vi "Monty_Hall_Game_Premium[1].vi"() -> ()   [LabVIEW 2025]
uses:
  <vilib>/numeric/Random Number (Range) I64.vi
  <vilib>/numeric/sub_Random U32.vi
panel:
  in  "Number of doors":i32=1 min=3 max=10 step=1
  out "Boolean 10":bool
  out "Boolean 9":bool
  out "Boolean 8":bool
  out "Boolean 7":bool
  out "Boolean 6":bool
  out "Boolean 5":bool
  out "Boolean 4":bool
  out "Boolean 3":bool
  out "Boolean 2":bool
  out "Boolean":bool
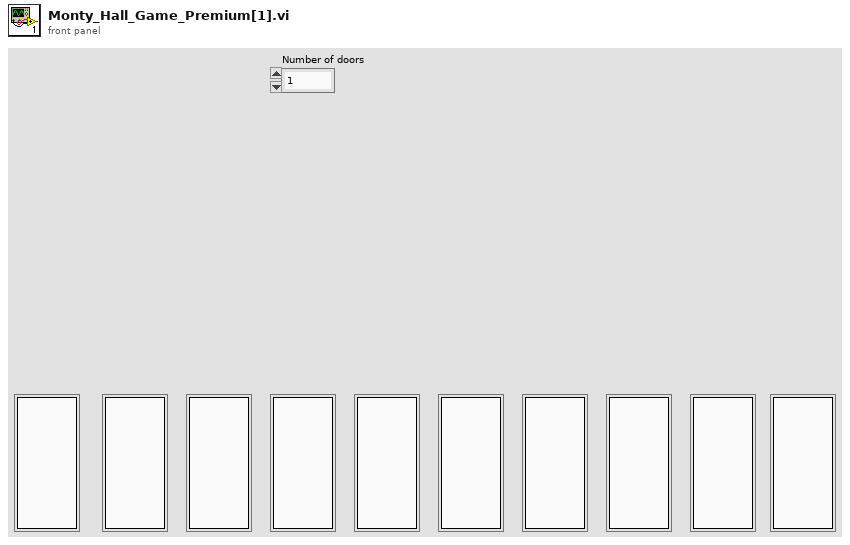
[diagram p1: front panel]
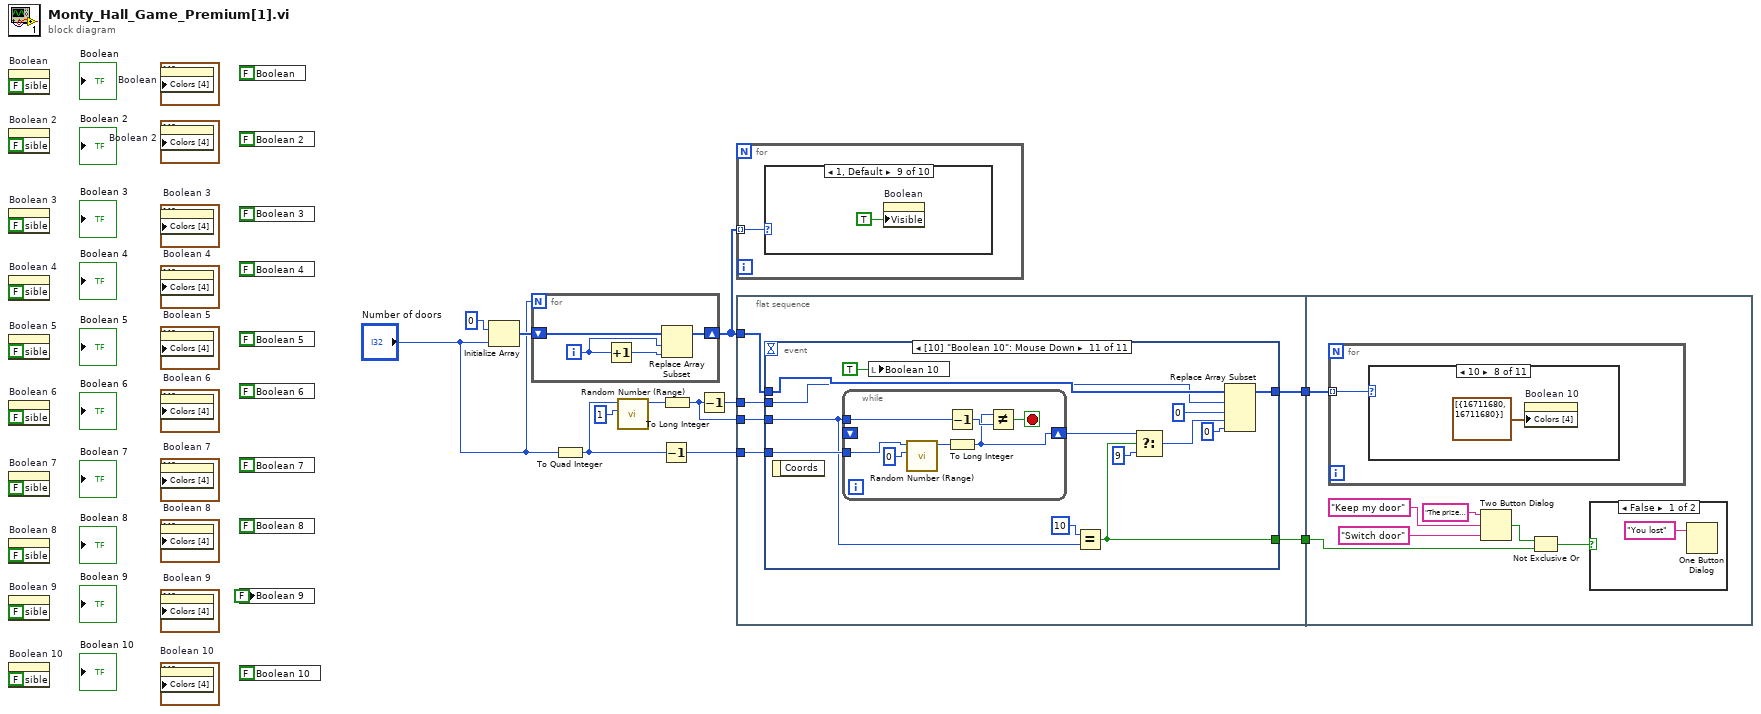
[diagram p0: block diagram]
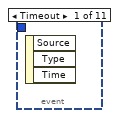
[diagram p2: hidden frame]
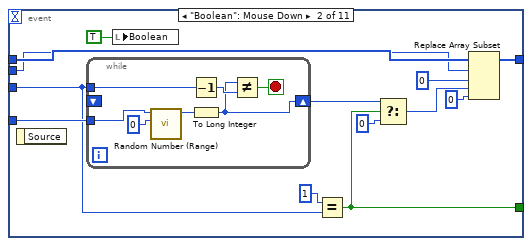
[diagram p3: hidden frame]
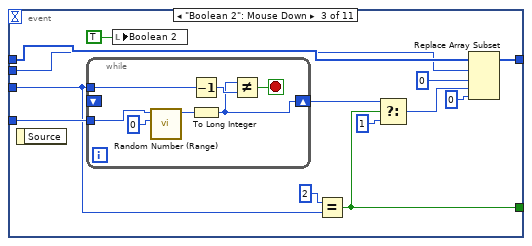
[diagram p4: hidden frame]
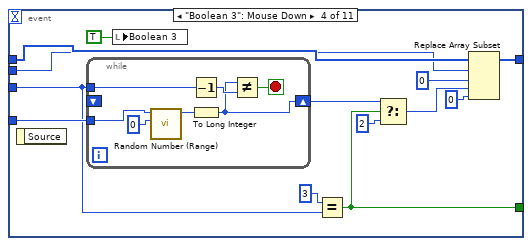
[diagram p5: hidden frame]
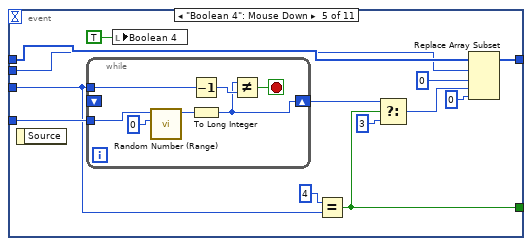
[diagram p6: hidden frame]
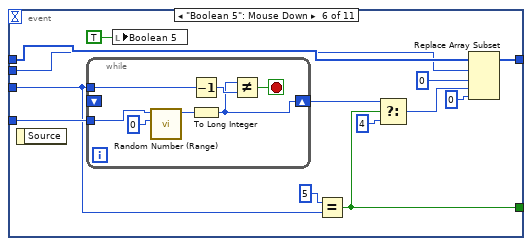
[diagram p7: hidden frame]
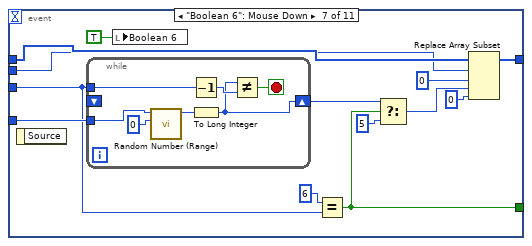
[diagram p8: hidden frame]
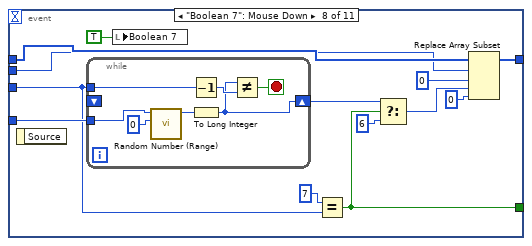
[diagram p9: hidden frame]
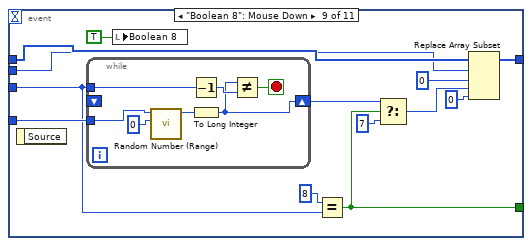
[diagram p10: hidden frame]
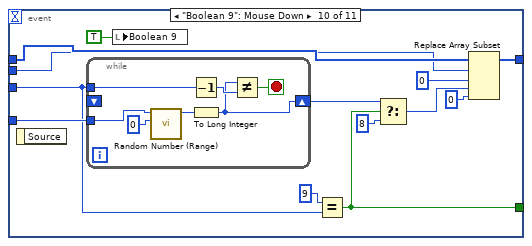
[diagram p11: hidden frame]
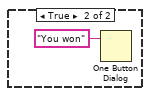
[diagram p12: hidden frame]
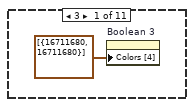
[diagram p13: hidden frame]
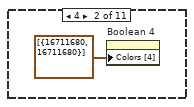
[diagram p14: hidden frame]
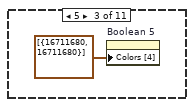
[diagram p15: hidden frame]
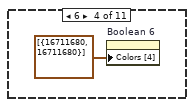
[diagram p16: hidden frame]
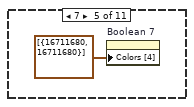
[diagram p17: hidden frame]
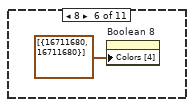
[diagram p18: hidden frame]
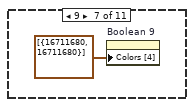
[diagram p19: hidden frame]
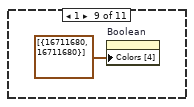
[diagram p20: hidden frame]
diagram:
  n1 = property on="Boolean" class="Bool (strict)"("Visible"=FALSE) -> ()  [unwired: 2 in, 2 out]
  n2 = property on="Boolean 2" class="Bool (strict)"("Visible"=FALSE) -> ()  [unwired: 2 in, 2 out]
  n3 = property on="Boolean 3" class="Bool (strict)"("Visible"=FALSE) -> ()  [unwired: 2 in, 2 out]
  n4 = property on="Boolean 4" class="Bool (strict)"("Visible"=FALSE) -> ()  [unwired: 2 in, 2 out]
  n5 = property on="Boolean 5" class="Bool (strict)"("Visible"=FALSE) -> ()  [unwired: 2 in, 2 out]
  n6 = property on="Boolean 6" class="Bool (strict)"("Visible"=FALSE) -> ()  [unwired: 2 in, 2 out]
  n7 = property on="Boolean 7" class="Bool (strict)"("Visible"=FALSE) -> ()  [unwired: 2 in, 2 out]
  n8 = property on="Boolean 8" class="Bool (strict)"("Visible"=FALSE) -> ()  [unwired: 2 in, 2 out]
  n9 = property on="Boolean 9" class="Bool (strict)"("Visible"=FALSE) -> ()  [unwired: 2 in, 2 out]
  n10 = property on="Boolean 10" class="Bool (strict)"("Visible"=FALSE) -> ()  [unwired: 2 in, 2 out]
  n11 = property on="Boolean" class="Bool (strict)"("Colors [4]"=cluster{u32, u32}[] [{0, 16448250}]) -> ()  [unwired: 2 in, 2 out]
  n12 = property on="Boolean 2" class="Bool (strict)"("Colors [4]"=cluster{u32, u32}[] [{0, 16448250}]) -> ()  [unwired: 2 in, 2 out]
  n13 = property on="Boolean 3" class="Bool (strict)"("Colors [4]"=cluster{u32, u32}[] [{0, 16448250}]) -> ()  [unwired: 2 in, 2 out]
  n14 = property on="Boolean 4" class="Bool (strict)"("Colors [4]"=cluster{u32, u32}[] [{0, 16448250}]) -> ()  [unwired: 2 in, 2 out]
  n15 = property on="Boolean 5" class="Bool (strict)"("Colors [4]"=cluster{u32, u32}[] [{0, 16448250}]) -> ()  [unwired: 2 in, 2 out]
  n16 = property on="Boolean 6" class="Bool (strict)"("Colors [4]"=cluster{u32, u32}[] [{0, 16448250}]) -> ()  [unwired: 2 in, 2 out]
  n17 = property on="Boolean 7" class="Bool (strict)"("Colors [4]"=cluster{u32, u32}[] [{0, 16448250}]) -> ()  [unwired: 2 in, 2 out]
  n18 = property on="Boolean 8" class="Bool (strict)"("Colors [4]"=cluster{u32, u32}[] [{0, 16448250}]) -> ()  [unwired: 2 in, 2 out]
  n19 = property on="Boolean 9" class="Bool (strict)"("Colors [4]"=cluster{u32, u32}[] [{0, 16448250}]) -> ()  [unwired: 2 in, 2 out]
  n20 = property on="Boolean 10" class="Bool (strict)"("Colors [4]"=cluster{u32, u32}[] [{0, 16448250}]) -> ()  [unwired: 2 in, 2 out]
  n21 = local write "Boolean"(FALSE ("Boolean")) -> ()
  n22 = local write "Boolean 2"(FALSE ("Boolean")) -> ()
  n23 = local write "Boolean 3"(FALSE ("Boolean")) -> ()
  n24 = local write "Boolean 4"(FALSE ("Boolean")) -> ()
  n25 = local write "Boolean 5"(FALSE ("Boolean")) -> ()
  n26 = local write "Boolean 6"(FALSE ("Boolean")) -> ()
  n27 = local write "Boolean 7"(FALSE ("Boolean")) -> ()
  n28 = local write "Boolean 8"(FALSE ("Boolean")) -> ()
  n29 = local write "Boolean 9"(FALSE ("Boolean")) -> ()
  n30 = local write "Boolean 10"(FALSE ("Boolean")) -> ()
  n31 = Initialize Array(0 ("element"), "Number of doors") -> (w41:i32[])
  n32 = for {
    N: "Number of doors" -> [_]
    shift-right: [w43] -> w28
    shift-left: w41 -> [w46]
    i -> [w45]
    n33 = Increment(x=w45) -> (x+1=w44:i32)
    n34 = Replace Array Subset(array=w46, new element=w44, index=w45) -> (w43:i32[])
  }
  n35 = To Quad Integer(1:"Number of doors") -> (0:w24:i64)
  n36 = call-poly <vilib>:"Random Number (Range).vi"("lower bound (-100)"=i64 1, "upper bound (100)"=w24) -> ("number"=w27:i64)  [unwired: 9 in]
  n37 = Decrement(x=w24) -> (x-1=w23:i64)
  n38 = To Long Integer(number=w27) -> (32bit integer=w26:i32)
  n39 = Decrement(x=w26) -> (x-1=w25:i32)
  n40 = for {
    tunnel: w28 -> [w47] mode=indexing
    n41 = case shown="1, Default" w47 {
      frame 3 {
        n42 = property on="Boolean 3" class="Bool (strict)"("Visible"=TRUE ("Boolean 4")) -> ()  [unwired: 2 in, 2 out]
      }
      frame 4 {
        n43 = property on="Boolean 4" class="Bool (strict)"("Visible"=TRUE) -> ()  [unwired: 2 in, 2 out]
      }
      frame 5 {
        n44 = property on="Boolean 5" class="Bool (strict)"("Visible"=TRUE) -> ()  [unwired: 2 in, 2 out]
      }
      frame 6 {
        n45 = property on="Boolean 6" class="Bool (strict)"("Visible"=TRUE) -> ()  [unwired: 2 in, 2 out]
      }
      frame 7 {
        n46 = property on="Boolean 7" class="Bool (strict)"("Visible"=TRUE) -> ()  [unwired: 2 in, 2 out]
      }
      frame 8 {
        n47 = property on="Boolean 8" class="Bool (strict)"("Visible"=TRUE) -> ()  [unwired: 2 in, 2 out]
      }
      frame 9 {
        n48 = property on="Boolean 9" class="Bool (strict)"("Visible"=TRUE) -> ()  [unwired: 2 in, 2 out]
      }
      frame 10 {
        n49 = property on="Boolean 10" class="Bool (strict)"("Visible"=TRUE) -> ()  [unwired: 2 in, 2 out]
      }
      frame 1, Default {
        n50 = property on="Boolean" class="Bool (strict)"("Visible"=TRUE) -> ()  [unwired: 2 in, 2 out]
      }
      frame 2 {
        n51 = property on="Boolean 2" class="Bool (strict)"("Visible"=TRUE ("Boolean 4")) -> ()  [unwired: 2 in, 2 out]
      }
    }
  }
  n52 = flat-sequence {
    tunnel: w28 -> [w63]
    tunnel: w26 -> [w62]
    tunnel: w25 -> [w61]
    tunnel: w23 -> [w60]
    tunnel: [w59] -> w22
    tunnel: [w58] -> w1
    tunnel: w22 -> [w270]
    tunnel: w1 -> [w267]
    frame #0 {
      n53 = event shown="[10] \"Boolean 10\": Mouse Down" {
        selector: _ -> [_ _ _ _ _ _ _ _ _ _ _]
        dyn-events: _ -> [_ _ _ _ _ _ _ _ _ _ _]
        timeout: _ -> [_ _ _ _ _ _ _ _ _ _ _]
        tunnel: w63 -> [_ w74 w90 w110 w130 w150 w170 w190 w210 w230 w250]
        tunnel: w62 -> [_ w69 w87 w107 w127 w147 w167 w187 w207 w227 w247]
        tunnel: w61 -> [_ w65 w89 w109 w129 w149 w169 w189 w209 w229 w249]
        tunnel: w60 -> [_ w70 w88 w108 w128 w148 w168 w188 w208 w228 w248]
        tunnel: [_ w67 w86 w106 w126 w146 w166 w186 w206 w226 w246] -> w59
        tunnel: [_ w64 w84 w104 w124 w144 w164 w184 w204 w224 w244] -> w58
        event Timeout {
          n54 = event-data() -> ()  [unwired: 1 in, 3 out]
        }
        event "Boolean": Mouse Down {
          n55 = event-data() -> ()  [unwired: 1 in, 1 out]
          n56 = while {
            tunnel: w70 -> [w81]
            tunnel: w69 -> [w79]
            shift-right: [w77] -> w68
            shift-left: _ -> [_]
            stop <- w78 stop-if-true
            n57 = call-poly <vilib>:"Random Number (Range).vi"("lower bound (-100)"=i64 0, "upper bound (100)"=w81) -> ("number"=w83:i64)  [unwired: 9 in]
            n58 = Decrement(x=w79) -> (x-1=w80:i32)
            n59 = To Long Integer(number=w83) -> (32bit integer=w77:i32)
            n60 = Not Equal?(x=w77, y=w80) -> (x != y?=w78:bool)
          }
          n61 = local write "Boolean"(TRUE ("Boolean")) -> ()
          n62 = Equal?(x=1, y=w69) -> (x = y?=w64:bool)
          n63 = Select(t=w68, s=w64, f=0 ("x")) -> (s? t:f=w72:i32)
          n64 = Replace Array Subset(array=w74, new element #1=0 ("new element/subarray"), index #1=w65, new element #2=0 ("new element/subarray"), index #2=w72) -> (w67:i32[])
        }
        event "Boolean 2": Mouse Down {
          n65 = event-data() -> ()  [unwired: 1 in, 1 out]
          n66 = while {
            tunnel: w88 -> [w101]
            tunnel: w87 -> [w99]
            shift-right: [w97] -> w91
            shift-left: _ -> [_]
            stop <- w98 stop-if-true
            n67 = call-poly <vilib>:"Random Number (Range).vi"("lower bound (-100)"=i64 0, "upper bound (100)"=w101) -> ("number"=w103:i64)  [unwired: 9 in]
            n68 = Decrement(x=w99) -> (x-1=w100:i32)
            n69 = To Long Integer(number=w103) -> (32bit integer=w97:i32)
            n70 = Not Equal?(x=w97, y=w100) -> (x != y?=w98:bool)
          }
          n71 = local write "Boolean 2"(TRUE ("Boolean")) -> ()
          n72 = Equal?(x=2, y=w87) -> (x = y?=w84:bool)
          n73 = Select(t=w91, s=w84, f=1 ("x")) -> (s? t:f=w93:i32)
          n74 = Replace Array Subset(array=w90, new element #1=0 ("new element/subarray"), index #1=w89, new element #2=0 ("new element/subarray"), index #2=w93) -> (w86:i32[])
        }
        event "Boolean 3": Mouse Down {
          n75 = event-data() -> ()  [unwired: 1 in, 1 out]
          n76 = while {
            tunnel: w108 -> [w121]
            tunnel: w107 -> [w119]
            shift-right: [w117] -> w111
            shift-left: _ -> [_]
            stop <- w118 stop-if-true
            n77 = call-poly <vilib>:"Random Number (Range).vi"("lower bound (-100)"=i64 0, "upper bound (100)"=w121) -> ("number"=w123:i64)  [unwired: 9 in]
            n78 = Decrement(x=w119) -> (x-1=w120:i32)
            n79 = To Long Integer(number=w123) -> (32bit integer=w117:i32)
            n80 = Not Equal?(x=w117, y=w120) -> (x != y?=w118:bool)
          }
          n81 = local write "Boolean 3"(TRUE ("Boolean")) -> ()
          n82 = Equal?(x=3, y=w107) -> (x = y?=w104:bool)
          n83 = Select(t=w111, s=w104, f=2 ("x")) -> (s? t:f=w113:i32)
          n84 = Replace Array Subset(array=w110, new element #1=0 ("new element/subarray"), index #1=w109, new element #2=0 ("new element/subarray"), index #2=w113) -> (w106:i32[])
        }
        event "Boolean 4": Mouse Down {
          n85 = event-data() -> ()  [unwired: 1 in, 1 out]
          n86 = while {
            tunnel: w128 -> [w141]
            tunnel: w127 -> [w139]
            shift-right: [w137] -> w131
            shift-left: _ -> [_]
            stop <- w138 stop-if-true
            n87 = call-poly <vilib>:"Random Number (Range).vi"("lower bound (-100)"=i64 0, "upper bound (100)"=w141) -> ("number"=w143:i64)  [unwired: 9 in]
            n88 = Decrement(x=w139) -> (x-1=w140:i32)
            n89 = To Long Integer(number=w143) -> (32bit integer=w137:i32)
            n90 = Not Equal?(x=w137, y=w140) -> (x != y?=w138:bool)
          }
          n91 = local write "Boolean 4"(TRUE ("Boolean")) -> ()
          n92 = Equal?(x=4, y=w127) -> (x = y?=w124:bool)
          n93 = Select(t=w131, s=w124, f=3 ("x")) -> (s? t:f=w133:i32)
          n94 = Replace Array Subset(array=w130, new element #1=0 ("new element/subarray"), index #1=w129, new element #2=0 ("new element/subarray"), index #2=w133) -> (w126:i32[])
        }
        event "Boolean 5": Mouse Down {
          n95 = event-data() -> ()  [unwired: 1 in, 1 out]
          n96 = while {
            tunnel: w148 -> [w161]
            tunnel: w147 -> [w159]
            shift-right: [w157] -> w151
            shift-left: _ -> [_]
            stop <- w158 stop-if-true
            n97 = call-poly <vilib>:"Random Number (Range).vi"("lower bound (-100)"=i64 0, "upper bound (100)"=w161) -> ("number"=w163:i64)  [unwired: 9 in]
            n98 = Decrement(x=w159) -> (x-1=w160:i32)
            n99 = To Long Integer(number=w163) -> (32bit integer=w157:i32)
            n100 = Not Equal?(x=w157, y=w160) -> (x != y?=w158:bool)
          }
          n101 = local write "Boolean 5"(TRUE ("Boolean")) -> ()
          n102 = Equal?(x=5, y=w147) -> (x = y?=w144:bool)
          n103 = Select(t=w151, s=w144, f=4 ("x")) -> (s? t:f=w153:i32)
          n104 = Replace Array Subset(array=w150, new element #1=0 ("new element/subarray"), index #1=w149, new element #2=0 ("new element/subarray"), index #2=w153) -> (w146:i32[])
        }
        event "Boolean 6": Mouse Down {
          n105 = event-data() -> ()  [unwired: 1 in, 1 out]
          n106 = while {
            tunnel: w168 -> [w181]
            tunnel: w167 -> [w179]
            shift-right: [w177] -> w171
            shift-left: _ -> [_]
            stop <- w178 stop-if-true
            n107 = call-poly <vilib>:"Random Number (Range).vi"("lower bound (-100)"=i64 0, "upper bound (100)"=w181) -> ("number"=w183:i64)  [unwired: 9 in]
            n108 = Decrement(x=w179) -> (x-1=w180:i32)
            n109 = To Long Integer(number=w183) -> (32bit integer=w177:i32)
            n110 = Not Equal?(x=w177, y=w180) -> (x != y?=w178:bool)
          }
          n111 = local write "Boolean 6"(TRUE ("Boolean")) -> ()
          n112 = Equal?(x=6, y=w167) -> (x = y?=w164:bool)
          n113 = Select(t=w171, s=w164, f=5 ("x")) -> (s? t:f=w173:i32)
          n114 = Replace Array Subset(array=w170, new element #1=0 ("new element/subarray"), index #1=w169, new element #2=0 ("new element/subarray"), index #2=w173) -> (w166:i32[])
        }
        event "Boolean 7": Mouse Down {
          n115 = event-data() -> ()  [unwired: 1 in, 1 out]
          n116 = while {
            tunnel: w188 -> [w201]
            tunnel: w187 -> [w199]
            shift-right: [w197] -> w191
            shift-left: _ -> [_]
            stop <- w198 stop-if-true
            n117 = call-poly <vilib>:"Random Number (Range).vi"("lower bound (-100)"=i64 0, "upper bound (100)"=w201) -> ("number"=w203:i64)  [unwired: 9 in]
            n118 = Decrement(x=w199) -> (x-1=w200:i32)
            n119 = To Long Integer(number=w203) -> (32bit integer=w197:i32)
            n120 = Not Equal?(x=w197, y=w200) -> (x != y?=w198:bool)
          }
          n121 = local write "Boolean 7"(TRUE ("Boolean")) -> ()
          n122 = Equal?(x=7, y=w187) -> (x = y?=w184:bool)
          n123 = Select(t=w191, s=w184, f=6 ("x")) -> (s? t:f=w193:i32)
          n124 = Replace Array Subset(array=w190, new element #1=0 ("new element/subarray"), index #1=w189, new element #2=0 ("new element/subarray"), index #2=w193) -> (w186:i32[])
        }
        event "Boolean 8": Mouse Down {
          n125 = event-data() -> ()  [unwired: 1 in, 1 out]
          n126 = while {
            tunnel: w208 -> [w221]
            tunnel: w207 -> [w219]
            shift-right: [w217] -> w211
            shift-left: _ -> [_]
            stop <- w218 stop-if-true
            n127 = call-poly <vilib>:"Random Number (Range).vi"("lower bound (-100)"=i64 0, "upper bound (100)"=w221) -> ("number"=w223:i64)  [unwired: 9 in]
            n128 = Decrement(x=w219) -> (x-1=w220:i32)
            n129 = To Long Integer(number=w223) -> (32bit integer=w217:i32)
            n130 = Not Equal?(x=w217, y=w220) -> (x != y?=w218:bool)
          }
          n131 = local write "Boolean 8"(TRUE ("Boolean")) -> ()
          n132 = Equal?(x=8, y=w207) -> (x = y?=w204:bool)
          n133 = Select(t=w211, s=w204, f=7 ("x")) -> (s? t:f=w213:i32)
          n134 = Replace Array Subset(array=w210, new element #1=0 ("new element/subarray"), index #1=w209, new element #2=0 ("new element/subarray"), index #2=w213) -> (w206:i32[])
        }
        event "Boolean 9": Mouse Down {
          n135 = event-data() -> ()  [unwired: 1 in, 1 out]
          n136 = while {
            tunnel: w228 -> [w241]
            tunnel: w227 -> [w239]
            shift-right: [w237] -> w231
            shift-left: _ -> [_]
            stop <- w238 stop-if-true
            n137 = call-poly <vilib>:"Random Number (Range).vi"("lower bound (-100)"=i64 0, "upper bound (100)"=w241) -> ("number"=w243:i64)  [unwired: 9 in]
            n138 = Decrement(x=w239) -> (x-1=w240:i32)
            n139 = To Long Integer(number=w243) -> (32bit integer=w237:i32)
            n140 = Not Equal?(x=w237, y=w240) -> (x != y?=w238:bool)
          }
          n141 = local write "Boolean 9"(TRUE ("Boolean")) -> ()
          n142 = Equal?(x=9, y=w227) -> (x = y?=w224:bool)
          n143 = Select(t=w231, s=w224, f=8 ("x")) -> (s? t:f=w233:i32)
          n144 = Replace Array Subset(array=w230, new element #1=0 ("new element/subarray"), index #1=w229, new element #2=0 ("new element/subarray"), index #2=w233) -> (w226:i32[])
        }
        event "Boolean 10": Mouse Down {
          n145 = event-data() -> ()  [unwired: 1 in, 1 out]
          n146 = while {
            tunnel: w248 -> [w261]
            tunnel: w247 -> [w259]
            shift-right: [w257] -> w251
            shift-left: _ -> [_]
            stop <- w258 stop-if-true
            n147 = call-poly <vilib>:"Random Number (Range).vi"("lower bound (-100)"=i64 0, "upper bound (100)"=w261) -> ("number"=w263:i64)  [unwired: 9 in]
            n148 = Decrement(x=w259) -> (x-1=w260:i32)
            n149 = To Long Integer(number=w263) -> (32bit integer=w257:i32)
            n150 = Not Equal?(x=w257, y=w260) -> (x != y?=w258:bool)
          }
          n151 = local write "Boolean 10"(TRUE ("Boolean")) -> ()
          n152 = Equal?(x=10, y=w247) -> (x = y?=w244:bool)
          n153 = Select(t=w251, s=w244, f=9 ("x")) -> (s? t:f=w253:i32)
          n154 = Replace Array Subset(array=w250, new element #1=0 ("new element/subarray"), index #1=w249, new element #2=0 ("new element/subarray"), index #2=w253) -> (w246:i32[])
        }
      }
    }
    frame #1 {
      n155 = for {
        tunnel: w270 -> [w273] mode=indexing
        n156 = case shown="10" w273 {
          frame 3 {
            n157 = property on="Boolean 3" class="Bool (strict)"("Colors [4]"=cluster{u32, u32}[] [{16711680, 16711680}]) -> ()  [unwired: 2 in, 2 out]
          }
          frame 4 {
            n158 = property on="Boolean 4" class="Bool (strict)"("Colors [4]"=cluster{u32, u32}[] [{16711680, 16711680}]) -> ()  [unwired: 2 in, 2 out]
          }
          frame 5 {
            n159 = property on="Boolean 5" class="Bool (strict)"("Colors [4]"=cluster{u32, u32}[] [{16711680, 16711680}]) -> ()  [unwired: 2 in, 2 out]
          }
          frame 6 {
            n160 = property on="Boolean 6" class="Bool (strict)"("Colors [4]"=cluster{u32, u32}[] [{16711680, 16711680}]) -> ()  [unwired: 2 in, 2 out]
          }
          frame 7 {
            n161 = property on="Boolean 7" class="Bool (strict)"("Colors [4]"=cluster{u32, u32}[] [{16711680, 16711680}]) -> ()  [unwired: 2 in, 2 out]
          }
          frame 8 {
            n162 = property on="Boolean 8" class="Bool (strict)"("Colors [4]"=cluster{u32, u32}[] [{16711680, 16711680}]) -> ()  [unwired: 2 in, 2 out]
          }
          frame 9 {
            n163 = property on="Boolean 9" class="Bool (strict)"("Colors [4]"=cluster{u32, u32}[] [{16711680, 16711680}]) -> ()  [unwired: 2 in, 2 out]
          }
          frame 10 {
            n164 = property on="Boolean 10" class="Bool (strict)"("Colors [4]"=cluster{u32, u32}[] [{16711680, 16711680}]) -> ()  [unwired: 2 in, 2 out]
          }
          frame 1 {
            n165 = property on="Boolean" class="Bool (strict)"("Colors [4]"=cluster{u32, u32}[] [{16711680, 16711680}]) -> ()  [unwired: 2 in, 2 out]
          }
          frame 0, Default {
          }
          frame 2 {
            n166 = property on="Boolean 2" class="Bool (strict)"("Colors [4]"=cluster{u32, u32}[] [{16711680, 16711680}]) -> ()  [unwired: 2 in, 2 out]
          }
        }
      }
      n167 = Two Button Dialog(message="The prize is not behind the red doors. Do you want to change your door ?", 1:"Switch door" ("T button name (\"OK\")"), 2:"Keep my door" ("F button name (\"Cancel\")")) -> (T button?=w268:bool)
      n168 = Not Exclusive Or(1:w267, 2:w268) -> (0:w264:bool)
      n169 = case shown="False" w264 {
        frame False {
          n170 = One Button Dialog(message="You lost") -> ()  [unwired: 1 in, 1 out]
        }
        frame True {
          n171 = One Button Dialog(message="You won") -> ()  [unwired: 1 in, 1 out]
        }
      }
    }
  }
